vi "MCList-Detect click on empty row.vi"(8 "error in (no error)":errorcluster, 9 "Coords":T2, 11 "MulticolumnListbox in":refnum<vi>) -> (0 "error out":errorcluster, 1 "Clicked on empty row":bool, 2 "Cell Position":T1, 3 "MulticolumnListbox out":refnum<vi>)   [LabVIEW 2020]
uses:
  <vilib>/Utility/miscctls.llb/LVPoint32TypeDef.ctl
  <vilib>/Utility/miscctls.llb/LVRowAndColumnTypeDef.ctl
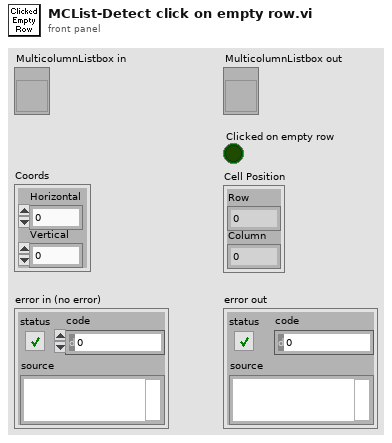
[diagram p1: front panel]
types:
  T1 = typedef "LVRowAndColumnTypeDef.ctl" = cluster{"Row":i32, "Column":i32}
  T2 = typedef "LVPoint32TypeDef.ctl" = cluster{"Horizontal":i32, "Vertical":i32}
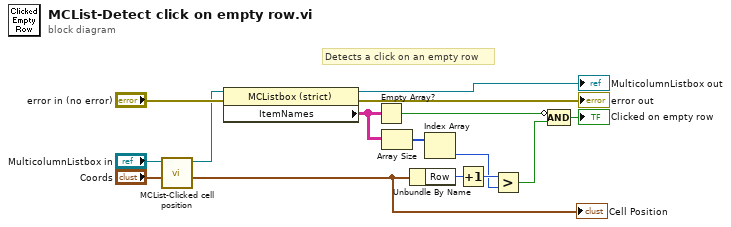
[diagram p0: block diagram]
diagram:
  # "Detects a click on an empty row"
  n1 = call "MCList-Clicked cell position.vi"("Coords"="Coords", "MulticolumnListbox in"="MulticolumnListbox in") -> ("Cell Position"=w1:T1, "MulticolumnListbox out"=w3:refnum<vi>)  [unwired: 8 in]
  "Cell Position" <- w1
  n2 = property class="MCListbox (strict)"(reference=w3, error in="error in (no error)") -> (reference out=→"MulticolumnListbox out":refnum<vi>, error out=→"error out":errorcluster, "ItemNames"=w12:string[][])
  n3 = Empty Array?(array=w12) -> (empty?=w13:bool)
  n4 = Array Size(array=w12) -> (size(s)=w15:i32[])
  n5 = Unbundle By Name(w1) -> ("Row"=w11:i32)
  n6 = Index Array(array=w15) -> (element=w9:i32)  [unwired: 1 in]
  n7 = Increment(x=w11) -> (x+1=w10:i32)
  n8 = Greater?(x=w10, y=w9) -> (0:w8:bool)
  n9 = Compound Arithmetic op=AND(invert w13, w8) -> (→"Clicked on empty row":bool)
